vi "Register Object in Selection.vi"(8 "error in":errorcluster, 10 "Object":refnum<vi>, 11 "Selection in":T1) -> (0 "error out":errorcluster, 2 "Owning Diag Ref":refnum<vi>, 3 "Selection out":T1, 4 "Owning Diag Already Registered?":bool, 5 "Owning Diag UID":i32)   [LabVIEW 2020, in "Enclose in Structure.lvlib"]
uses:
  Enclose in Structure.lvlib
  <vilib>/Utility/miscctls.llb/LVMapReplaceAction.ctl
  Selection Map.ctl
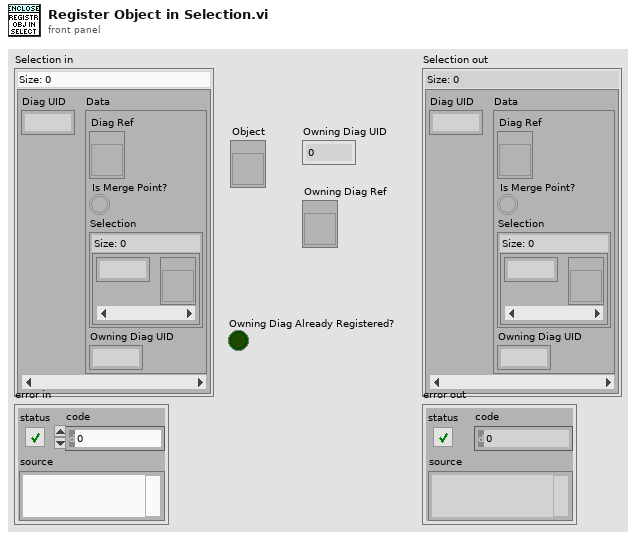
[diagram p1: front panel]
types:
  T1 = typedef "Enclose in Structure.lvlib/Selection Map.ctl" = map{i32, cluster{"Diag Ref":refnum<vi>, "Is Merge Point?":bool, "Selection":map{i32, refnum<vi>}, "Owning Diag UID":i32}}
  T2 = typedef "LVMapReplaceAction.ctl" = enum32{"Modify Entry only if found", "Add or Modify Entry", "Delete Entry"}
  T3 = cluster{"Diag Ref":refnum<vi>, "Is Merge Point?":bool, "Selection":map{i32, refnum<vi>}, "Owning Diag UID":i32}
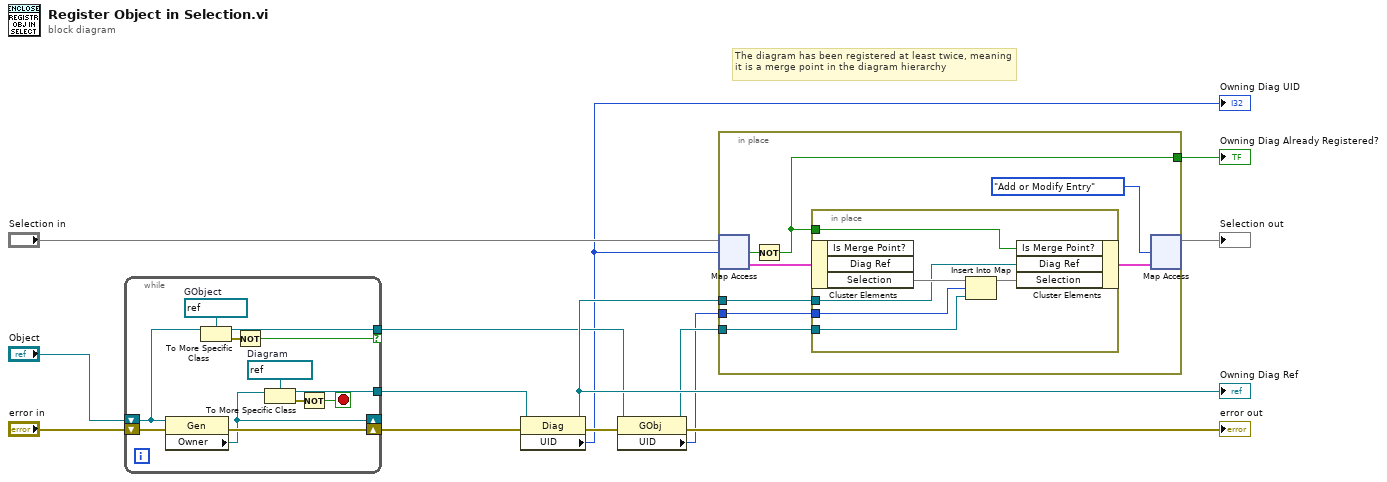
[diagram p0: block diagram]
diagram:
  # "The diagram has been registered at least twice, meaning it is a merge point in the diagram hierarchy"
  n1 = while {
    shift-right: [w17] -> _
    shift-left: "Object" -> [w19]
    tunnel: [w24] -> w4 if=w23
    tunnel: [w18] -> w6
    shift-right: [w26] -> w12
    shift-left: "error in" -> [w16]
    stop <- w15 stop-if-true
    w20 = refnum<vi> refnum  # Diagram
    w25 = refnum<vi> refnum  # GObject
    n2 = property class="Gen"(reference=w19, error in=w16) -> (error out=w26:errorcluster, "Owner"=w17:refnum<vi>)  [unwired: 1 out]
    n3 = To More Specific Class(target class=w25, reference=w19) -> (specific class reference=w24:refnum<vi>, error out=w22:errorcluster)  [unwired: 1 in]
    n4 = Not(x=w22) -> (.not. x?=w23:bool)
    n5 = To More Specific Class(target class=w20, reference=w17) -> (specific class reference=w18:refnum<vi>, error out=w21:errorcluster)  [unwired: 1 in]
    n6 = Not(x=w21) -> (.not. x?=w15:bool)
  }
  n7 = property class="Diag"(reference=w6, error in=w12) -> (reference out=w5:refnum<vi>, error out=w11:errorcluster, "UID"=w2:i32)
  "Owning Diag UID" <- w2
  "Owning Diag Ref" <- w5
  n8 = property class="GObj"(reference=w4, error in=w11) -> (reference out=w3:refnum<vi>, error out=→"error out":errorcluster, "UID"=w1:i32)
  n9 = in-place {
    in-place-border: w1 -> [w33]
    in-place-border: w5 -> [w30]
    in-place-border: w3 -> [w29]
    in-place-border: [w27] -> w7
    n10 = in-place-map #1("Selection in", w2) -> (w32:T3, w28:bool)  [unwired: 1 in]
    n11 = Not(x=w28) -> (.not. x?=w27:bool)
    n12 = in-place {
      in-place-border: w33 -> [w38]
      in-place-border: w30 -> [w36]
      in-place-border: w29 -> [w37]
      in-place-border: w27 -> [w35]
      n13 = in-place-cluster #2(w32) -> ("Selection"=w40:map{i32, refnum<vi>})  [unwired: 2 out]
      n14 = Insert Into Map(map in=w40, key=w38, value=w37) -> (map out=w39:map{i32, refnum<vi>})  [unwired: 2 out]
      n15 = in-place-cluster #2("Is Merge Point?"=w35, "Diag Ref"=w36, "Selection"=w39) -> (w31:T3)
    }
    n16 = in-place-map #1(w31, LVMapReplaceAction."Add or Modify Entry" ("action")) -> (→"Selection out":T1)  [unwired: 2 out]
  }
  "Owning Diag Already Registered?" <- w7
